vi "Transceiver.Initialize.vi"(8 "error in (no error)":errorcluster, 9 "transceiver settings":T1, 10 "Transfer Groups Configurations":refnum<class "Transfer Group Configuration.lvclass">[](array[class]), 11 "Transceiver in":refnum<class "Transceiver.lvclass">) -> (0 "error out":errorcluster, 3 "Transceiver out":refnum<class "Transceiver.lvclass">)   [LabVIEW 2017, in "DSF.Engine.lvlib" / "Transceiver.lvclass"]
uses:
  Transceiver.lvclass
  Shared/Classes/Transfer Group/Transfer Group Configuration.lvclass
  DSF Configuration API/1.0.0/Public/Controls/DSF Settings Info.ctl
  DSF Configuration API/1.0.0/DSF Configuration API.lvlib
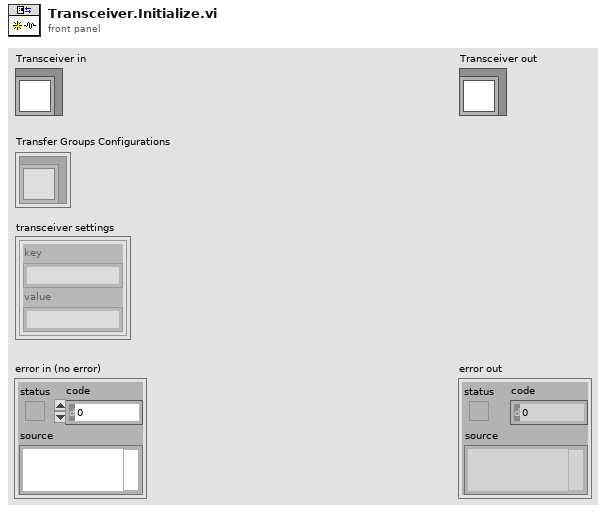
[diagram p1: front panel]
types:
  T1 = typedef "DSF Configuration API.lvlib/DSF Settings Info.ctl" = cluster{"key":string, "value":string}[]
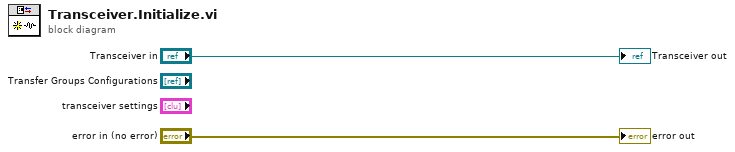
[diagram p0: block diagram]
diagram:
  "error out" <- "error in (no error)"
  "Transceiver out" <- "Transceiver in"
